vi "SET_DEVICE_MEASURE_TO_GLOBAL.vi"(6 "TRIGGER":bool=TRUE, 9 "DEVICE in":string, 11 "USB_DEV":string) -> (2 "DEVICE? 2":bool, 3 "JSON string response 2":string)   [LabVIEW 2015]
uses:
  Share Data/uPower_kit.ctl
panel:
  in  "DEV_BUSY":T1
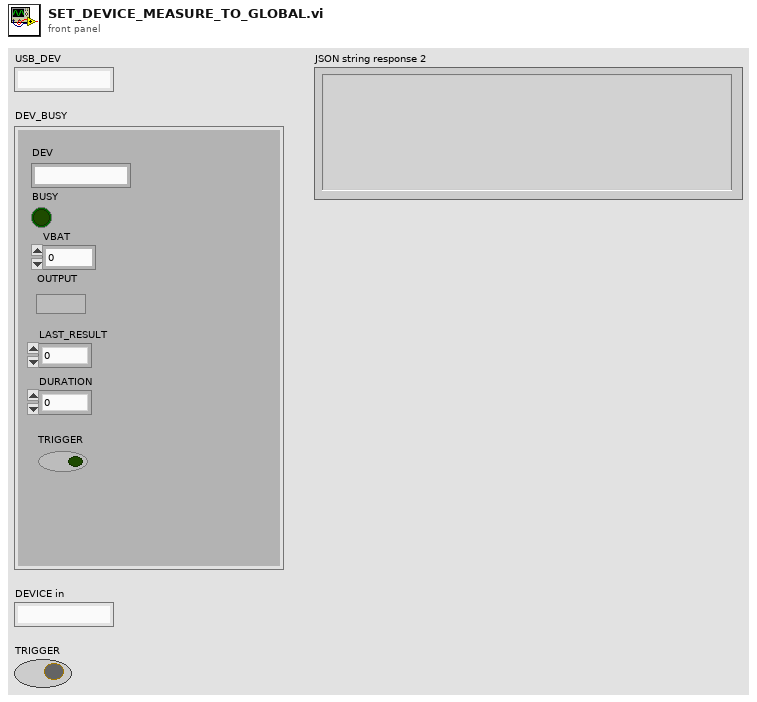
[diagram p1: front panel]
types:
  T1 = typedef "uPower_kit.ctl" = cluster{"DEV":string, "BUSY":bool, "VBAT":dbl, "OUTPUT":bool, "LAST_RESULT":dbl, "DURATION":dbl, "TRIGGER":bool}
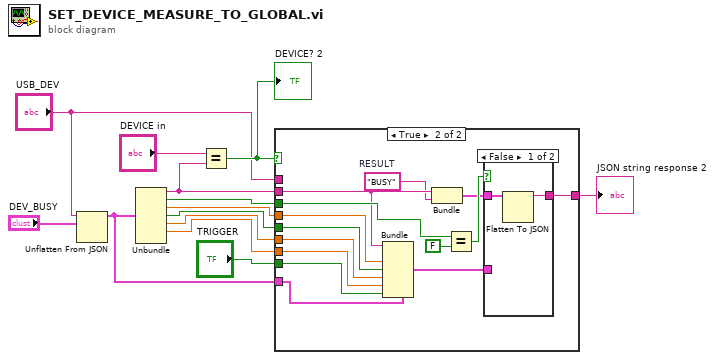
[diagram p0: block diagram]
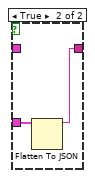
[diagram p3: hidden frame]
diagram:
  n1 = Unflatten From JSON(JSON string="USB_DEV", type and defaults="DEV_BUSY") -> (value=w9:T1)  [unwired: 5 in, 1 out]
  n2 = Unbundle(w9) -> ("DEV"=w6:string, "BUSY"=w5:bool, "VBAT"=w4:dbl, "OUTPUT"=w3:bool, "LAST_RESULT"=w2:dbl, "DURATION"=w12:dbl)  [unwired: 1 out]
  n3 = Equal?(x="DEVICE in", y=w6) -> (x = y?=w7:bool)
  "DEVICE? 2" <- w7
  n4 = case shown="True" w7 {
    tunnel: w9 -> [_ w28]
    tunnel: w6 -> [_ w17]
    tunnel: w5 -> [_ w20]
    tunnel: w4 -> [_ w21]
    tunnel: w3 -> [_ w22]
    tunnel: w2 -> [_ w27]
    tunnel: [w14 w25] -> w11
    tunnel: "USB_DEV" -> [w14 _]
    tunnel: w12 -> [_ w24]
    tunnel: "TRIGGER" -> [_ w23]
    frame False {
    }
    frame True {
      w16 = "BUSY"  # RESULT
      n5 = Bundle(cluster=w28, "DEV"=w17, "VBAT"=w21, "OUTPUT"=w22, "LAST_RESULT"=w27, "DURATION"=w24, "TRIGGER"=w23) -> (w26:T1)  [unwired: 1 in]
      n6 = Bundle("DEV"=w17, "RESULT"=w16) -> (w15:cluster{"DEV":string, "RESULT":string})  [unwired: 1 in]
      n7 = Equal?(x=w20, y=FALSE) -> (x = y?=w18:bool)
      n8 = case shown="False" w18 {
        tunnel: w26 -> [_ w32]
        tunnel: [w29 w31] -> w25
        tunnel: w15 -> [w30 _]
        frame False {
          n9 = Flatten To JSON(anything=w30) -> (JSON string=w29:string)  [unwired: 2 in, 1 out]
        }
        frame True {
          n10 = Flatten To JSON(anything=w32) -> (JSON string=w31:string)  [unwired: 2 in, 1 out]
        }
      }
    }
  }
  "JSON string response 2" <- w11
